vi "subImage_CenterAroundRoi.vi"(1 "ROI in":T1={"Bin"=1, "ROI"={"x offset"=0, "y offset"=0, "x width"=2048, "y width"=2048}} caption="Current" {"ROI"."x offset" min=1 max=512 step=1; "ROI"."y offset" min=1 max=512 step=1; "ROI"."x width" min=1 max=512 step=1; "ROI"."y width" min=1 max=512 step=1; "Bin" items=["1x1"=1, "2x2"=2, "4x4"=4]}) -> (0 "Graph scale":T2={"X min"=0, "Y min"=0, "X max"=2048, "Y max"=2048} {"X min" min=1 max=512 step=1; "Y min" min=1 max=512 step=1; "X max" min=1 max=512 step=1; "Y max" min=1 max=512 step=1})   [LabVIEW 2015]
panel:
  # "Center graph scale round ROI"
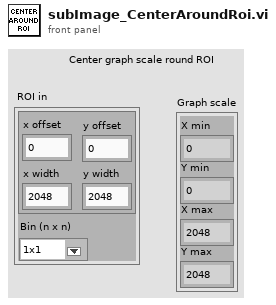
[diagram p1: front panel]
types:
  T1 = cluster{"Bin":u16, "ROI":cluster{"x offset":i32, "y offset":i32, "x width":i32, "y width":i32}}
  T2 = cluster{"X min":i32, "Y min":i32, "X max":i32, "Y max":i32}
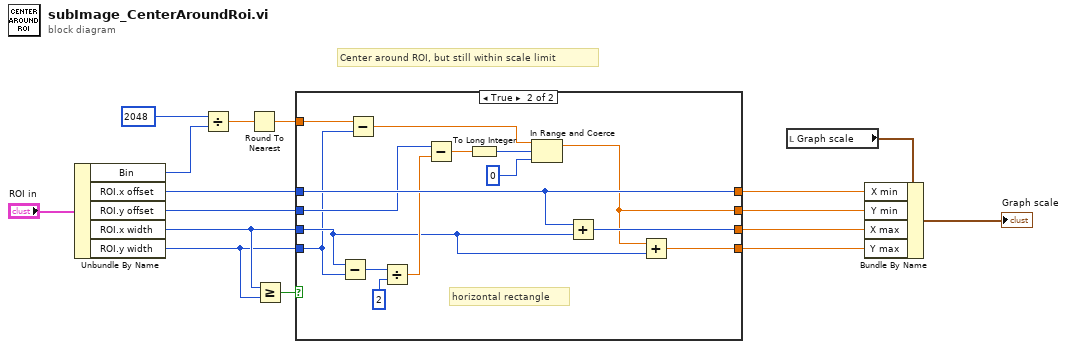
[diagram p0: block diagram]
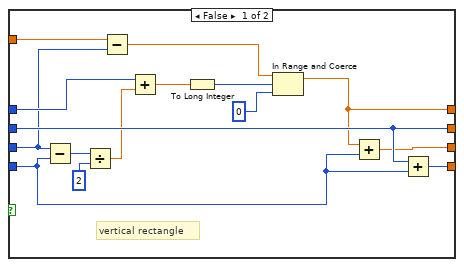
[diagram p2: hidden frame]
diagram:
  # "Center around ROI, but still within scale limit"
  n1 = Unbundle By Name("ROI in") -> ("Bin"=w5:u16, "ROI.x offset"=w4:i32, "ROI.y offset"=w3:i32, "ROI.x width"=w2:i32, "ROI.y width"=w1:i32)
  n2 = Divide(x=2048 ("Binned pixels"), y=w5) -> (x/y=w8:dbl)
  n3 = Round To Nearest(number=w8) -> (nearest integer value=w7:dbl)
  n4 = Greater Or Equal?(x=w2, y=w1) -> (x >= y?=w16:bool)
  n5 = case shown="True" w16 {
    tunnel: w2 -> [w20 w37]
    tunnel: w1 -> [w24 w35]
    tunnel: w3 -> [w30 w44]
    tunnel: w4 -> [w27 w45]
    tunnel: [w19 w45] -> w15
    tunnel: [w25 w46] -> w13
    tunnel: [w30 w34] -> w14
    tunnel: [w31 w40] -> w12
    tunnel: w7 -> [w22 w36]
    frame False {
      # "vertical rectangle"
      n6 = Subtract(x=w20, y=w24) -> (x-y=w29:i32)
      n7 = Divide(x=w29, y=u16 2 ("element")) -> (x/y=w26:dbl)
      n8 = Subtract(x=w22, y=w20) -> (x-y=w21:dbl)
      n9 = Add(x=w27, y=w26) -> (x+y=w18:dbl)
      n10 = To Long Integer(number=w18) -> (32bit integer=w17:i32)
      n11 = In Range and Coerce(upper limit=w21, x=w17, lower limit=0) -> (coerced(x)=w19:dbl)  [unwired: 1 out]
      n12 = Add(x=w19, y=w24) -> (x+y=w25:dbl)
      n13 = Add(x=w30, y=w24) -> (x+y=w31:i32)
    }
    frame True {
      # "horizontal rectangle"
      n14 = Subtract(x=w37, y=w35) -> (x-y=w43:i32)
      n15 = Subtract(x=w36, y=w35) -> (x-y=w38:dbl)
      n16 = Divide(x=w43, y=u16 2 ("element")) -> (x/y=w41:dbl)
      n17 = Subtract(x=w44, y=w41) -> (x-y=w33:dbl)
      n18 = To Long Integer(number=w33) -> (32bit integer=w32:i32)
      n19 = In Range and Coerce(upper limit=w38, x=w32, lower limit=0) -> (coerced(x)=w34:dbl)  [unwired: 1 out]
      n20 = Add(x=w45, y=w37) -> (x+y=w46:i32)
      n21 = Add(x=w34, y=w37) -> (x+y=w40:dbl)
    }
  }
  n22 = local read "Graph scale"() -> (w10:T2)
  n23 = Bundle By Name(cluster=w10, "X min"=w15, "Y min"=w14, "X max"=w13, "Y max"=w12) -> (→"Graph scale":T2)
